vi "Read Switches V.5.0.vi"   [LabVIEW 2016]
uses:
  Robot Global Data V.5.0.vi
  <vilib>/Rock Robotics/Network Tables/NT Read Boolean.vi
types:
  T1 = typedef "WPI_SwitchDevRef.ctl" = cluster{"DevStatus":errorcluster, "DIO Channel":T2, "CntIndex":T3, "Normally Closed":bool}
  T2 = typedef "FPGA_DIOChannel.ctl" = enum8{"DIO 0", "DIO 1", "DIO 2", "DIO 3", "DIO 4", "DIO 5", "DIO 6", "DIO 7", "DIO 8", "DIO 9", "DIO MXP 0", "DIO MXP 1", "DIO MXP 2", "DIO MXP 3", "DIO MXP 4", "DIO MXP 5", "DIO MXP 6", "DIO MXP 7", "DIO MXP 8", "DIO MXP 9", "DIO MXP 10", "DIO MXP 11", "DIO MXP 12", "DIO MXP 13", "DIO MXP 14", "DIO MXP 15", "SPI Port CS1", "SPI Port CS2", "SPI Port CS3", "SPI Port MISO", "SPI Port MOSI", "Invalid"}
  T3 = typedef "FPGA_CounterCtrSystemIndex.ctl" = enum8{"Ctr 0", "Ctr 1", "Ctr 2", "Ctr 3", "Ctr 4", "Ctr 5", "Ctr 6", "Ctr 7", "Invalid"}
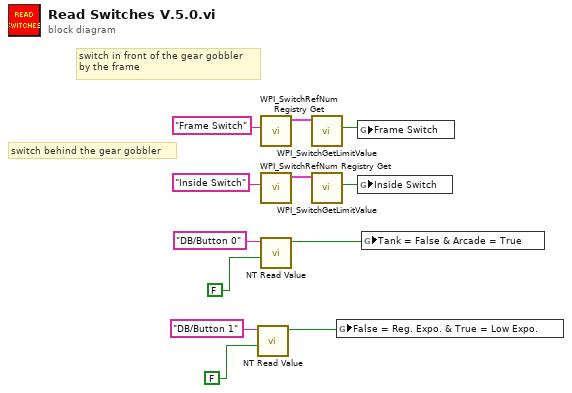
[diagram p0: block diagram]
diagram:
  # "switch behind the gear gobbler"
  # "switch in front of the gear gobbler\nby the frame"
  n1 = call-poly <vilib>:"NT Read Value.vi"("Default Value"=FALSE, "Name"="DB/Button 1" ("refnum name")) -> ("Boolean"=w2:bool)  [unwired: 8 in, 1 out]
  n2 = call <vilib>:"WPI_SwitchRefNum Registry Get.vi"("refnum name"="Frame Switch") -> ("SwitchDevRef"=w7:T1)  [unwired: 9 in, 1 out]
  n3 = call <vilib>:"WPI_SwitchRefNum Registry Get.vi"("refnum name"="Inside Switch") -> ("SwitchDevRef"=w9:T1)  [unwired: 9 in, 1 out]
  n4 = call-poly <vilib>:"NT Read Value.vi"("Default Value"=FALSE, "Name"="DB/Button 0" ("refnum name")) -> ("Boolean"=w11:bool)  [unwired: 8 in, 1 out]
  n5 = call <vilib>:"WPI_SwitchGetLimitValue.vi"("SwitchDevRef"=w7) -> ("Switch Pressed"=w6:bool)  [unwired: 8 in, 2 out]
  n6 = call <vilib>:"WPI_SwitchGetLimitValue.vi"("SwitchDevRef"=w9) -> ("Switch Pressed"=w5:bool)  [unwired: 8 in, 2 out]
  n7 = global write "Robot Global Data V.5.0.vi" "False = Reg. Expo. & True = Low Expo."(w2) -> ()
  n8 = global write "Robot Global Data V.5.0.vi" "Frame Switch"(w6) -> ()
  n9 = global write "Robot Global Data V.5.0.vi" "Inside Switch"(w5) -> ()
  n10 = global write "Robot Global Data V.5.0.vi" "Tank = False & Arcade = True"(w11) -> ()
